vi "Flywheel_Execute.vi"() -> ()   [LabVIEW 2019]
uses:
  <vilib>/Rock Robotics/WPI/ThirdParty/REV Robotics/SPARK MAX/Typedef/Spark MAX Control Type.ctl
  Globals/Flywheel_Globals.vi
panel:
  in  "Ramp Rate Auto":sgl
  in  "Ramp Rate Manual":sgl=5.0
  in  "Max Speed":dbl=5100.0
  out "Sensor Velocity":dbl
  # "Click here to set min"
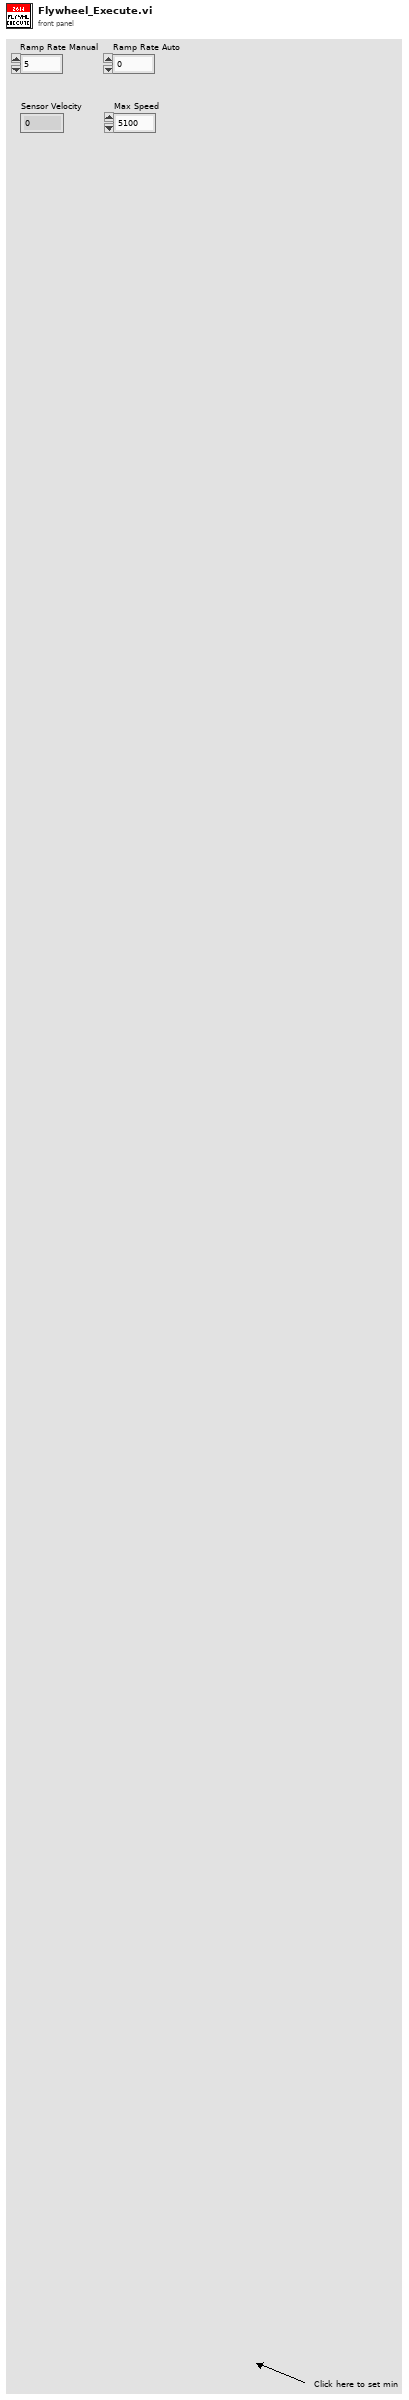
[diagram p1: front panel]
types:
  T1 = typedef "WPI_MotorControlDeviceRef.ctl" = cluster{"DeviceStatus":errorcluster, "Type":T2, "PWM":cluster{"PWM Channel":T3, "DeadBand":T4}, "CAN":cluster{"Device Number":u8, "SetOutput VI Ref":variant, "GetOutput VI Ref":variant, "Enable VI Ref":variant, "Disable VI Ref":variant, "Data":variant}, "Invert":bool, "DIO PWM":cluster{"PWM \"Enable\" Channel":T3, "DIOChannel":T5, "PWM Rate":dbl}}
  T2 = typedef "WPI_MotorControlType.ctl" = enum16{"PWM", "CAN", "DIO PWM"}
  T3 = typedef "FPGA_DIOPWMChannel.ctl" = enum8{"PWM 0", "PWM 1", "PWM 2", "PWM 3", "PWM 4", "PWM 5", "PWM 6", "PWM 7", "PWM 8", "PWM 9", "PWM MXP 0", "PWM MXP 1", "PWM MXP 2", "PWM MXP 3", "PWM MXP 4", "PWM MXP 5", "PWM MXP 6", "PWM MXP 7", "PWM MXP 8", "PWM MXP 9", "Invalid"}
  T4 = typedef "WPI_PWMDeadband.ctl" = cluster{"Name":string, "maxPositivePwm":i32, "minPositivePwm":i32, "centerPwm":i32, "maxNegativePwm":i32, "minNegativePwm":i32, "angularRange":u16}
  T5 = typedef "FPGA_DIOChannel.ctl" = enum8{"DIO 0", "DIO 1", "DIO 2", "DIO 3", "DIO 4", "DIO 5", "DIO 6", "DIO 7", "DIO 8", "DIO 9", "DIO MXP 0", "DIO MXP 1", "DIO MXP 2", "DIO MXP 3", "DIO MXP 4", "DIO MXP 5", "DIO MXP 6", "DIO MXP 7", "DIO MXP 8", "DIO MXP 9", "DIO MXP 10", "DIO MXP 11", "DIO MXP 12", "DIO MXP 13", "DIO MXP 14", "DIO MXP 15", "SPI Port CS1", "SPI Port CS2", "SPI Port CS3", "SPI Port MISO", "SPI Port MOSI", "Invalid"}
  T6 = typedef "Spark MAX Control Type.ctl" = enum16{"Percent VBus", "Voltage", "Velocity", "Position", "Smart Motion", "Current", "Smart Velocity"}
  T7 = typedef "Flywheel_Cluster.ctl" = cluster{"Flywheel_Throttle":dbl, "Control_States":T8, "Auto_Speed":bool, "Flywheel_On":bool}
  T8 = typedef "Flywheel_States.ctl" = enum16{"No-Op", "Percent_Voltage", "Speed_Control_Manual", "Speed_Control_Auto"}
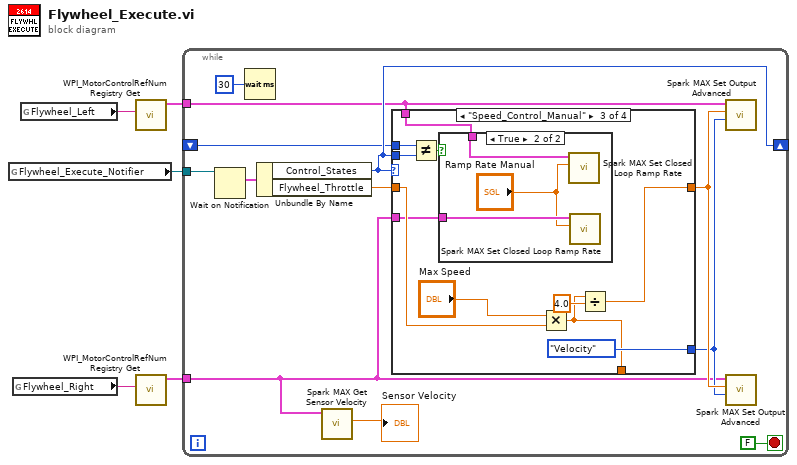
[diagram p0: block diagram]
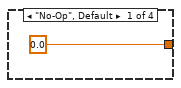
[diagram p2: hidden frame]
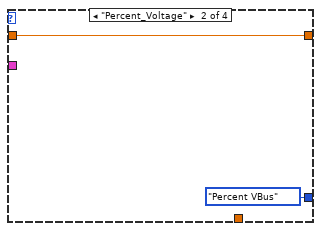
[diagram p3: hidden frame]
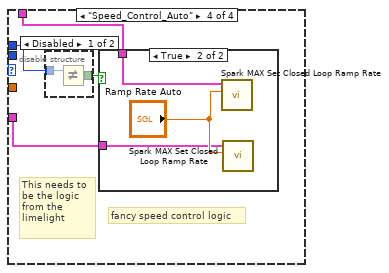
[diagram p5: hidden frame]
diagram:
  n1 = global read "Flywheel_Globals.vi" "Flywheel_Execute_Notifier"() -> (w5:refnum<notifier>)
  n2 = global read "Flywheel_Globals.vi" "Flywheel_Right"() -> (w4:string)
  n3 = global read "Flywheel_Globals.vi" "Flywheel_Left"() -> (w3:string)
  n4 = call <vilib>:"WPI_MotorControlRefNum Registry Get.vi"("refnum name"=w3) -> ("MotorControlDevRef"=w2:T1)  [unwired: 9 in, 1 out]
  n5 = call <vilib>:"WPI_MotorControlRefNum Registry Get.vi"("refnum name"=w4) -> ("MotorControlDevRef"=w1:T1)  [unwired: 9 in, 1 out]
  n6 = while {
    tunnel: w5 -> [w16]
    tunnel: w2 -> [w8]
    tunnel: w1 -> [w7]
    shift-right: [w10] -> _
    shift-left: _ -> [w9]
    stop <- FALSE stop-if-true
    n7 = Wait on Notification(notifier=w16) -> (notification=w15:T7)  [unwired: 3 in, 3 out]
    n8 = Wait (ms)(milliseconds to wait=u32 30) -> ()  [unwired: 1 out]
    n9 = Unbundle By Name(w15) -> ("Control_States"=w10:T8, "Flywheel_Throttle"=w14:dbl)
    n10 = call <vilib>:"Spark MAX Get Sensor Velocity.vi"("MotorControlDevRef in"=w7) -> ("Sensor Velocity"=→"Sensor Velocity":dbl)  [unwired: 7 in, 3 out]
    n11 = case shown="\"Speed_Control_Manual\"" w10 {
      tunnel: [0.0 ("Flywheel_Throttle") w20 w22 _] -> w12
      tunnel: w14 -> [_ w20 w29 _]
      tunnel: [_ Spark_MAX_Control_Type."Percent VBus" ("Control Mode") Spark_MAX_Control_Type."Velocity" ("Control Mode") _] -> w11
      tunnel: w10 -> [_ _ w28 _]
      tunnel: w9 -> [_ _ w27 w37]
      tunnel: w8 -> [_ _ w25 w36]
      tunnel: w7 -> [_ _ w24 w35]
      tunnel: [_ _ w21 _] -> _
      frame "No-Op", Default {
      }
      frame "Percent_Voltage" {
      }
      frame "Speed_Control_Manual" {
        n12 = Not Equal?(x=w27, y=w28) -> (x != y?=w26:bool)
        n13 = case shown="True" w26 {
          tunnel: w25 -> [_ w34]
          tunnel: w24 -> [_ w33]
          frame False {
          }
          frame True {
            n14 = call <vilib>:"Spark MAX Set Closed Loop Ramp Rate.vi"("Seconds from neutral to full (0)"="Ramp Rate Manual", "MotorControlDeviceRef in"=w34) -> ()  [unwired: 8 in, 2 out]
            n15 = call <vilib>:"Spark MAX Set Closed Loop Ramp Rate.vi"("Seconds from neutral to full (0)"="Ramp Rate Manual", "MotorControlDeviceRef in"=w33) -> ()  [unwired: 8 in, 2 out]
          }
        }
        n16 = Multiply(x="Max Speed", y=w29) -> (x*y=w21:dbl)
        n17 = Divide(x=w21, y=4.0) -> (x/y=w22:dbl)
      }
      frame "Speed_Control_Auto" {
        # "This needs to \nbe the logic \nfrom the \nlimelight"
        # "fancy speed control logic"
        n18 = disable-structure shown="Disabled" {
          disable-tunnel: [w40 _] -> w38
          disable-tunnel: w37 -> [w39 _]
          frame Disabled {
            n19 = Not Equal?(x=w39) -> (x != y?=w40:bool)  [unwired: 1 in]
          }
          frame Enabled {
          }
        }
        n20 = case shown="True" w38 {
          tunnel: w36 -> [_ w42]
          tunnel: w35 -> [_ w41]
          frame False {
          }
          frame True {
            n21 = call <vilib>:"Spark MAX Set Closed Loop Ramp Rate.vi"("Seconds from neutral to full (0)"="Ramp Rate Auto", "MotorControlDeviceRef in"=w42) -> ()  [unwired: 8 in, 2 out]
            n22 = call <vilib>:"Spark MAX Set Closed Loop Ramp Rate.vi"("Seconds from neutral to full (0)"="Ramp Rate Auto", "MotorControlDeviceRef in"=w41) -> ()  [unwired: 8 in, 2 out]
          }
        }
      }
    }
    n23 = call <vilib>:"Spark MAX Set Output Advanced.vi"("Control Mode"=w11, "Setpoint"=w12, "MotorControlDevRef"=w8) -> ()  [unwired: 7 in, 2 out]
    n24 = call <vilib>:"Spark MAX Set Output Advanced.vi"("Control Mode"=w11, "Setpoint"=w12, "MotorControlDevRef"=w7) -> ()  [unwired: 7 in, 2 out]
  }
